vi "Save_SpectralRepetitive.vi"(0 "Refnum in":refnum<k34>, 2 "Capture number":i32, 5 "New File":bool=TRUE, 7 "Image":dbl[][](array[numeric]), 11 "error in (no error)":errorcluster, 12 "Gate Delay":dbl, 13 "Wavelength Array":dbl[](array[numeric])) -> (4 "Refnum out":refnum<k34>, 15 "error out":errorcluster)   [LabVIEW 2017]
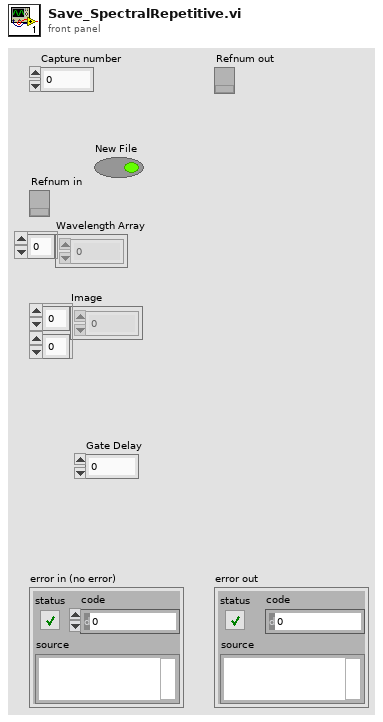
[diagram p1: front panel]
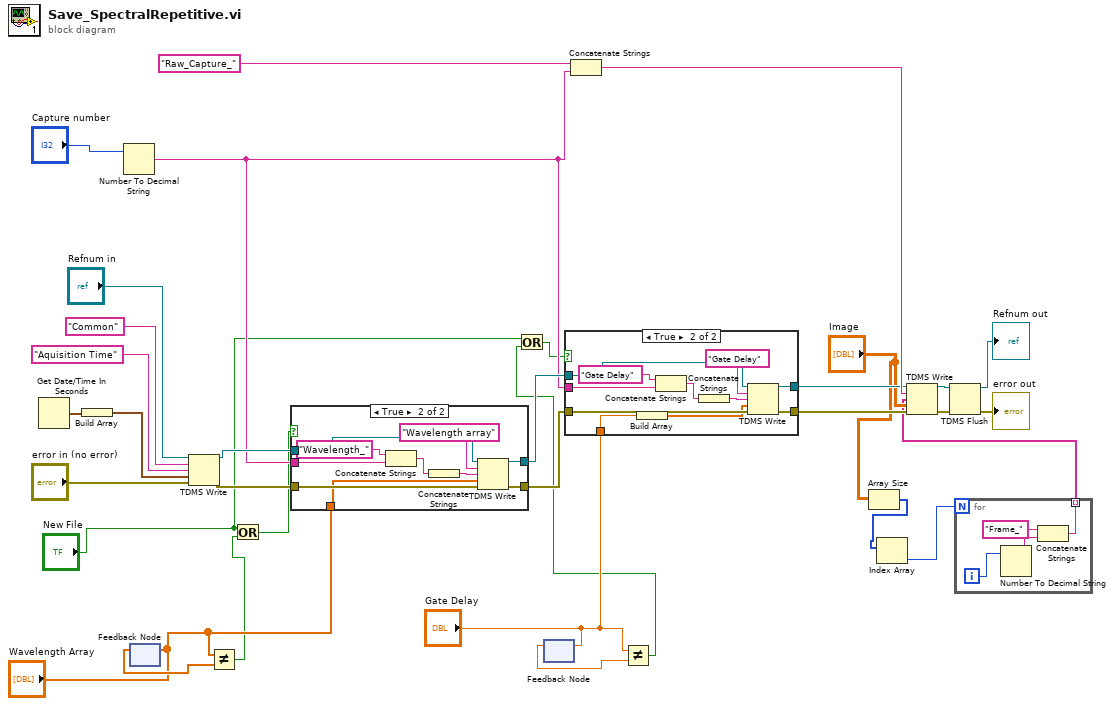
[diagram p0: block diagram]
diagram:
  n1 = Get Date/Time In Seconds() -> (seconds since 1Jan1904=w17:timestamp)
  n2 = Build Array(w17) -> (w21:timestamp[])
  n3 = Number To Decimal String(number="Capture number") -> (decimal integer string=w6:string)  [unwired: 1 in]
  n4 = feedback #1() -> (w8:dbl[])  [unwired: 1 in]
  n5 = feedback-in #1("Wavelength Array") -> ()
  n6 = TDMS Write(0:"Refnum in", 5:"Common" ("group name in (Untitled)"), 7:"Aquisition Time", 9:w21, 11:"error in (no error)") -> (4:w12:refnum<k34>, 15:w11:errorcluster)  [unwired: 1 in, 2 out]
  n7 = Not Equal?(x="Wavelength Array", y=w8) -> (x != y?=w5:bool)
  n8 = Or(x="New File", y=w5) -> (x .or. y?=w4:bool)
  n9 = case shown="True" w4 {
    tunnel: w12 -> [w35 w45]
    tunnel: w11 -> [w34 w44]
    tunnel: [w35 w43] -> w10
    tunnel: [w34 w42] -> w9
    tunnel: "Wavelength Array" -> [_ w39]
    tunnel: w6 -> [_ w36]
    frame False {
    }
    frame True {
      n10 = Concatenate Strings("Wavelength_" ("string"), w36) -> (w38:string)
      n11 = Concatenate Strings(w38) -> (w40:string)
      n12 = TDMS Write(0:w45, 5:"Wavelength array" ("group name in (Untitled)"), 7:w40, 9:w39, 11:w44) -> (4:w43:refnum<k34>, 15:w42:errorcluster)  [unwired: 1 in, 2 out]
    }
  }
  n13 = feedback #2() -> (w19:dbl)  [unwired: 1 in]
  n14 = feedback-in #2("Gate Delay") -> ()
  n15 = Concatenate Strings("Raw_Capture_" ("group name in (Untitled)"), w6) -> (w28:string)
  n16 = Not Equal?(x="Gate Delay", y=w19) -> (x != y?=w3:bool)
  n17 = Or(x="New File", y=w3) -> (x .or. y?=w1:bool)
  n18 = case shown="True" w1 {
    tunnel: w10 -> [w47 w58]
    tunnel: w9 -> [w46 w57]
    tunnel: [w47 w56] -> w23
    tunnel: [w46 w55] -> w24
    tunnel: "Gate Delay" -> [_ w49]
    tunnel: w6 -> [_ w50]
    frame False {
    }
    frame True {
      n19 = Build Array(w49) -> (w48:dbl[])
      n20 = Concatenate Strings("Gate Delay" ("string"), w50) -> (w52:string)
      n21 = Concatenate Strings(w52) -> (w53:string)
      n22 = TDMS Write(0:w58, 5:"Gate Delay" ("group name in (Untitled)"), 7:w53, 9:w48, 11:w57) -> (4:w56:refnum<k34>, 15:w55:errorcluster)  [unwired: 1 in, 2 out]
    }
  }
  n23 = Array Size(array="Image") -> (size(s)=w15:i32[])
  n24 = Index Array(array=w15) -> (element=w14:i32)  [unwired: 1 in]
  n25 = for {
    N: w14 -> [_]
    tunnel: [w59] -> w13 mode=indexing
    i -> [w62]
    n26 = Number To Decimal String(number=w62) -> (decimal integer string=w61:string)  [unwired: 1 in]
    n27 = Concatenate Strings("Frame_" ("string"), w61) -> (w59:string)
  }
  n28 = TDMS Write(0:w23, 5:w28, 7:w13, 9:"Image", 11:w24) -> (4:w25:refnum<k34>, 15:w26:errorcluster)  [unwired: 1 in, 2 out]
  n29 = TDMS Flush(4:w26, 7:w25) -> (0:→"error out":errorcluster, 3:→"Refnum out":refnum<k34>)
